vi "Fetch Trace.vi"(7 "Points":u32, 8 "error in (no error)":errorcluster, 9 "Trace":u16(ring) items=["Trace A", "Trace B", "Trace C", "Trace D", "Trace E"], 10 "Maximum time":u32=10000, 11 "VISA resource name":refnum<visa-resource-name>) -> (0 "error out":errorcluster, 1 "Y array":dbl[](array[numeric]), 2 "X array":dbl[](array[numeric]), 3 "VISA resource name out":refnum<visa-resource-name>)   [LabVIEW 2021, in "Ceyear.lvlib"]
doc: "Returns the acquired trace and scaling information from the spectrum analyzer. The trace is from an acquisition that you initiate prior to calling this VI. You initiate an acquisition with the <b>Initiate</b> VI.\n\n<B>Note:</B> \n\nUse this VI only with other low-level VIs. The high-level VIs automatically incorporate this functionality. This VI does not check the instrument status."
uses:
  <instrlib>/Ceyear/Ceyear.lvlib
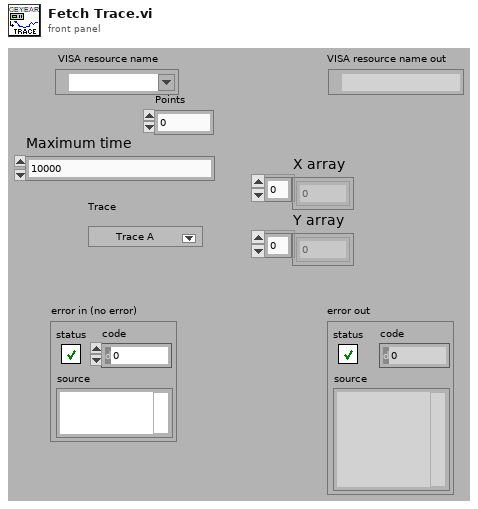
[diagram p1: front panel]
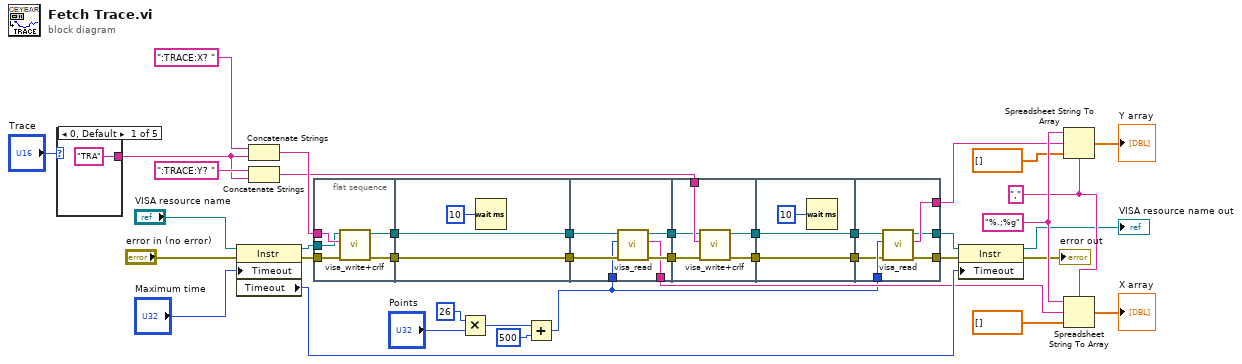
[diagram p0: block diagram]
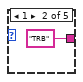
[diagram p2: hidden frame]
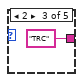
[diagram p3: hidden frame]
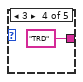
[diagram p4: hidden frame]
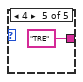
[diagram p5: hidden frame]
diagram:
  w35 = "," ("delimiter (Tab)")
  w36 = "%.;%g"
  n1 = case shown="0, Default" "Trace" {
    tunnel: ["TRA" "TRB" "TRC" "TRD" "TRE"] -> w1
    frame 0, Default {
    }
    frame 1 {
    }
    frame 2 {
    }
    frame 3 {
    }
    frame 4 {
    }
  }
  n2 = property class="Instr"(reference="VISA resource name", error in="error in (no error)", "Timeout"="Maximum time") -> (reference out=w22:refnum<visa-resource-name>, error out=w24:errorcluster, "Timeout"=w21:u32)
  n3 = Concatenate Strings(":TRACE:X? ", w1) -> (w23:string)
  n4 = Concatenate Strings(":TRACE:Y? ", w1) -> (w20:string)
  n5 = flat-sequence {
    tunnel: w24 -> [w47]
    tunnel: w23 -> [w49]
    tunnel: w22 -> [w48]
    tunnel: [w46] -> w13
    tunnel: [w45] -> w12
    tunnel: w13 -> [w52]
    tunnel: w12 -> [w51]
    tunnel: [w52] -> w11
    tunnel: [w51] -> w10
    tunnel: [w55] -> w16
    tunnel: [w53] -> w15
    tunnel: w11 -> [w58]
    tunnel: w8 -> [w57]
    tunnel: w10 -> [w56]
    tunnel: [w54] -> w9
    tunnel: w16 -> [w61]
    tunnel: w20 -> [w63]
    tunnel: w15 -> [w62]
    tunnel: [w60] -> w6
    tunnel: [w59] -> w5
    tunnel: [w66] -> w7
    tunnel: w6 -> [w66]
    tunnel: w5 -> [w65]
    tunnel: [w65] -> w4
    tunnel: [w69] -> w17
    tunnel: [w70] -> w18
    tunnel: [w71] -> w19
    tunnel: w8 -> [w72]
    tunnel: w7 -> [w68]
    tunnel: w4 -> [w67]
    frame #0 {
      n6 = call <instrlib>:"visa_write+crlf.vi"("error in (no error)"=w47, "Strings (empty)"=w49, "VISA resource name"=w48) -> ("error out"=w46:errorcluster, "VISA resource name out"=w45:refnum<visa-resource-name>)  [unwired: 7 in]
    }
    frame #1 {
      n7 = Wait (ms)(milliseconds to wait=u32 10) -> ()  [unwired: 1 out]
    }
    frame #2 {
      n8 = call <instrlib>:"visa_read.vi"("error in (no error)"=w58, "Byte Count (0)"=w57, "VISA resource name"=w56) -> ("error out"=w55:errorcluster, "Read Data"=w54:string, "VISA resource name out"=w53:refnum<visa-resource-name>)  [unwired: 5 in, 1 out]
    }
    frame #3 {
      n9 = call <instrlib>:"visa_write+crlf.vi"("error in (no error)"=w61, "Strings (empty)"=w63, "VISA resource name"=w62) -> ("error out"=w59:errorcluster, "VISA resource name out"=w60:refnum<visa-resource-name>)  [unwired: 7 in]
    }
    frame #4 {
      n10 = Wait (ms)(milliseconds to wait=u32 10) -> ()  [unwired: 1 out]
    }
    frame #5 {
      n11 = call <instrlib>:"visa_read.vi"("error in (no error)"=w67, "Byte Count (0)"=w72, "VISA resource name"=w68) -> ("error out"=w71:errorcluster, "Read Data"=w70:string, "VISA resource name out"=w69:refnum<visa-resource-name>)  [unwired: 5 in, 1 out]
    }
  }
  n12 = Multiply(x=u32 26 ("byte count"), y="Points") -> (x*y=w26:u32)
  n13 = Add(x=w26, y=u32 500) -> (x+y=w8:u32)
  n14 = property class="Instr"(reference=w17, error in=w19, "Timeout"=w21) -> (reference out=→"VISA resource name out":refnum<visa-resource-name>, error out=→"error out":errorcluster)
  n15 = Spreadsheet String To Array(delimiter (Tab)=w35, format string=w36, spreadsheet string=w18, array type (2D Dbl)=dbl[] []) -> (array=→"Y array":dbl[])
  n16 = Spreadsheet String To Array(delimiter (Tab)=w35, format string=w36, spreadsheet string=w9, array type (2D Dbl)=dbl[] []) -> (array=→"X array":dbl[])
